vi "0-Load Map.vi"(0 "Image Path":path) -> (1 "Image Out":T1, 2 "Image Descriptor":T2={"Upper-Left Corner Coordinates"={"UTM Zone"=0.0, "Hemisphere"=enum."North", "East"=0.0, "North"=0.0}, "Meters/Pixel"=1.0})   [LabVIEW 2011]
doc: "Loads a map and its corresponding descriptor text file from the given path. The image and the descriptor file must have the same filename (but different extensions - descriptor file is .txt)."
uses:
  0-Image Descriptor.ctl
  2-Think/2 Typedefs/UTM Location.ctl
  <vilib>/vision/Image Controls.llb/IMAQ Image.ctl
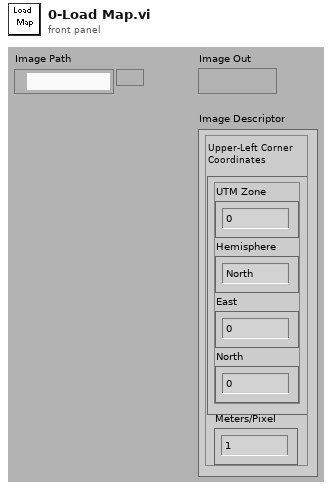
[diagram p1: front panel]
types:
  T1 = typedef "IMAQ Image.ctl" = refnum<image>
  T2 = typedef "0-Image Descriptor.ctl" = cluster{"Upper-Left Corner Coordinates":T3, "Meters/Pixel":dbl}
  T3 = typedef "UTM Location.ctl" = cluster{"UTM Zone":dbl, "Hemisphere":enum16{"North", "South"}, "East":dbl, "North":dbl}
  T4 = typedef "Image Type" = u32
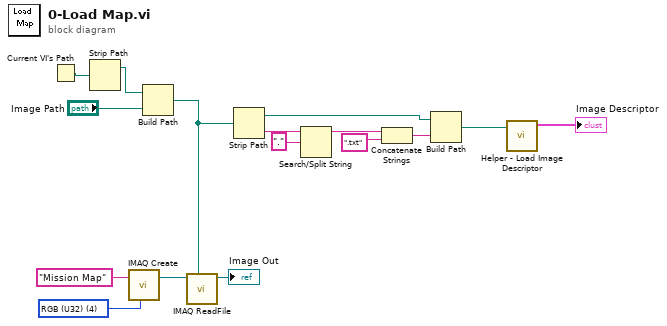
[diagram p0: block diagram]
diagram:
  w15 = T4 4 items=["Grayscale (U8)", "Grayscale (I16)", "Grayscale (SGL)", "Complex (CSG)", "RGB (U32)", "HSL (U32)", "RGB (U64)", "Grayscale (U16)"] ("Image Type")
  n1 = Current VI's Path() -> (path=w10:path)
  n2 = Strip Path(path=w10) -> (stripped path=w9:path)  [unwired: 1 out]
  n3 = call "IMAQ Create"("Image Name"="Mission Map", "Image Type"=w15) -> ("New Image"=w14:T1)  [unwired: 2 in, 2 out]
  n4 = Build Path(base path=w9, name or relative path="Image Path") -> (appended path=w2:path)
  n5 = call "IMAQ ReadFile"("File Path"=w2, "Image"=w14) -> ("Image Out"=→"Image Out":T1)  [unwired: 3 in, 6 out]
  n6 = Strip Path(path=w2) -> (stripped path=w4:path, name=w5:string)
  n7 = Search/Split String(string=w5, search string/char (-)=".") -> (substring before match=w6:string)  [unwired: 3 out]
  n8 = Concatenate Strings(w6, ".txt" ("string")) -> (w8:string)
  n9 = Build Path(base path=w4, name or relative path=w8) -> (appended path=w3:path)
  n10 = call "Helper - Load Image Descriptor.vi"("Image Descriptor File Path"=w3) -> ("Image Descriptor Typedef out"=→"Image Descriptor":T2)  [unwired: 10 in]
